vi "Create chemtrac files.vi"() -> ()   [LabVIEW 2019]
panel:
  in  "ChemTracChannels":string[](array[string])=["UV 1.1 UVA", "UV 1.1 UVT", "UV 1.1 Compensated UVA", "UV 1.1 COD", "UV 1.1 TOC", "PC 1.2 Cell ", "PC 1.2 Laser ", "PC 1.2 Total N", "PC 1.2 Bin 1 N", "PC 1.2 Bin 2 N", "PC 1.2 Bin 3 N", "PC 1.2 Bin 4 N", "PC 1.2 Bin 5 N", "PC 1.2 Bin 6 N", "PC 1.2 Total ppb", "PC 1.2 Bin 1 ppb", "PC 1.2 Bin 2 ppb", "PC 1.2 Bin 3 ppb", "PC 1.2 Bin 4 ppb", "PC 1.2 Bin 5 ppb", "PC 1.2 Bin 6 ppb", "PC 1.3 Cell ", "PC 1.3 Laser ", "PC 1.3 Total N", "PC 1.3 Bin 1 N", "PC 1.3 Bin 2 N", "PC 1.3 Bin 3 N", "PC 1.3 Bin 4 N", "PC 1.3 Bin 5 N", "PC 1.3 Bin 6 N", "PC 1.3 Total ppb", "PC 1.3 Bin 1 ppb", "PC 1.3 Bin 2 ppb", "PC 1.3 Bin 3 ppb", "PC 1.3 Bin 4 ppb", "PC 1.3 Bin 5 ppb", "PC 1.3 Bin 6 ppb"]
  in  "template path":path=path "C:/Users/mw24/Documents/GitHub/LabVIEW/ProCoDA/Control code/Modbus devices/Chemtrac/ChemTrac.vit"
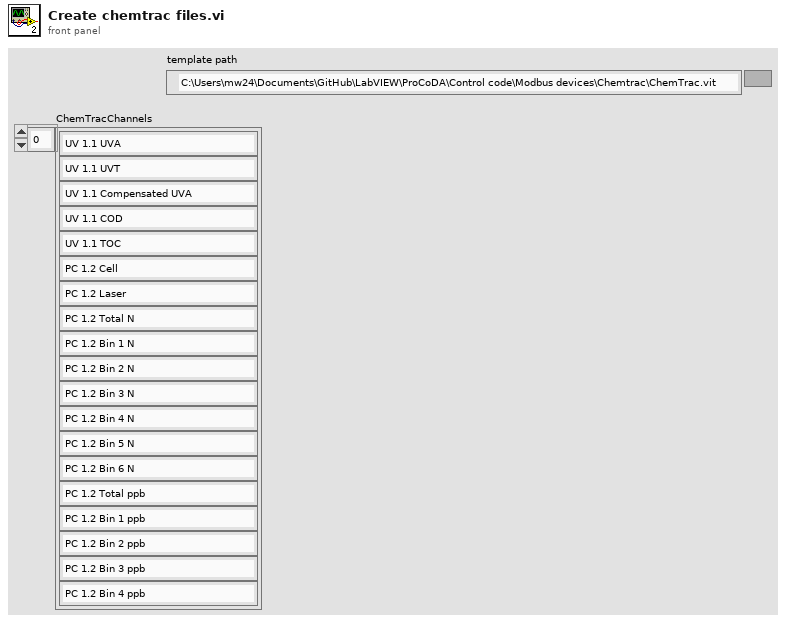
[diagram p1: front panel]
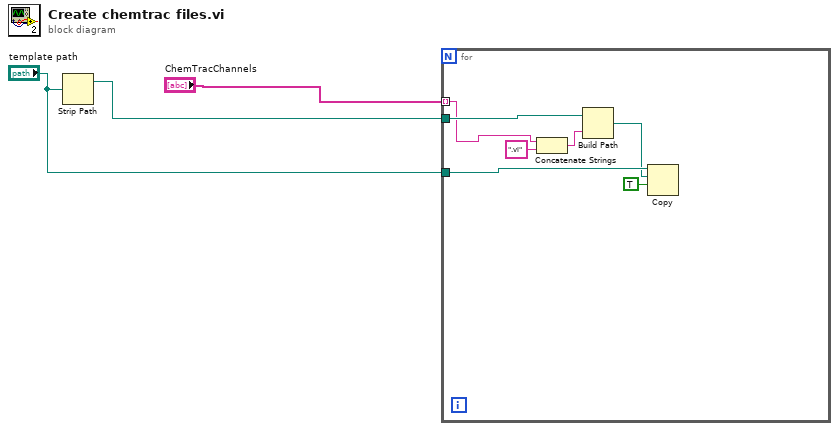
[diagram p0: block diagram]
diagram:
  n1 = Strip Path(path="template path") -> (stripped path=w2:path)  [unwired: 1 out]
  n2 = for {
    tunnel: "template path" -> [w10]
    tunnel: "ChemTracChannels" -> [w4] mode=indexing
    tunnel: w2 -> [w9]
    n3 = Concatenate Strings(w4, ".vi" ("string")) -> (w7:string)
    n4 = Build Path(base path=w9, name or relative path=w7) -> (appended path=w6:path)
    n5 = Copy(9:TRUE ("overwrite (F)"), 10:w6, 11:w10) -> ()  [unwired: 2 in, 3 out]
  }
